vi "fgt init Ex.vi"(8 "error in (no error)":errorcluster, 11 "SN":u16[](array[numeric])=array[4097 elements]) -> (0 "error out":errorcluster, 3 "SN out":u16[](array[numeric]))   [LabVIEW 2020, in "fgt_SDK.lvlib"]
doc: "Initialize specific Fluigent instrument(s) from their unique serial number. This function can be used when multiple instruments are connected in order to select your device(s)"
uses:
  fgt_SDK.lvlib
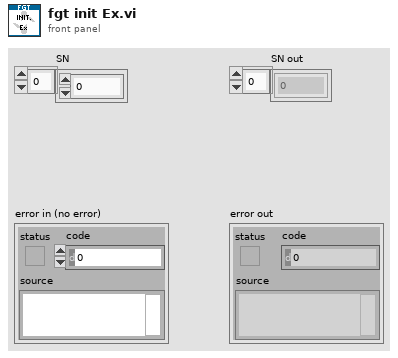
[diagram p1: front panel]
types:
  T1 = typedef "fgt_SDK.lvlib/fgt_STATUS_INFO.ctl" = cluster{"InstrType":T2, "instrSN":u16, "errorCode":u8, "infoCode":u8, "detail":string}
  T2 = typedef "fgt_SDK.lvlib/fgt_INSTRUMENT_TYPE.ctl" = enum32{"None", "MFCS", "MFCS_EZ", "FRP", "LineUP", "IPS"}
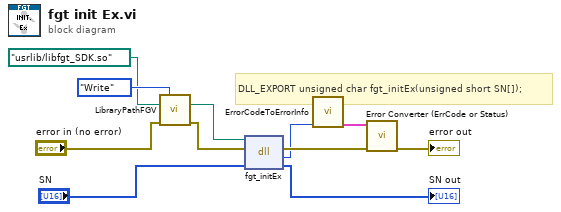
[diagram p0: block diagram]
diagram:
  # "DLL_EXPORT unsigned char fgt_initEx(unsigned short SN[]);"
  n1 = call "LibraryPathFGV.vi"("Action"=enum16{"Read", "Write"}."Write", "Path In"=path "/usrlib/libfgt_SDK.so", "error in (no error)"="error in (no error)") -> ("Path Out"=w1:path, "error out"=w2:errorcluster)  [unwired: 11 in]
  n2 = dll-call lib="C:/Workspace/fgt-SDK/LabVIEW/dlls/fgt_SDK_*.*" fn="fgt_initEx"(path in=w1, error in=w2, "SN"="SN") -> (error out=w9:errorcluster, "return type"=w7:u8, "SN"=→"SN out":u16[])  [unwired: 1 in, 1 out]
  n3 = call "ErrorCodeToErrorInfo.vi"("return type"=w7) -> ("StatusInfo"=w6:T1)  [unwired: 10 in]
  n4 = call "Error Converter (ErrCode or Status).vi"("error in (no error)"=w9, "StatusInfo"=w6) -> ("error out"=→"error out":errorcluster)  [unwired: 9 in]
